vi "Find Average BP Center.vi"(7 "Tray Number":i32, 9 "XYZTheta":dbl[](array[numeric]), 11 "Gantry In":refnum<k24>) -> (1 "XYZTheta Centers":dbl[][](array[numeric]), 3 "Gantry Out":refnum<k24>)   [LabVIEW 2019, in "Assembly Tray.lvclass"]
uses:
  Assembly Tray.lvclass
  Controller/Camera/Machine Vision.ctl
  C:/Program Files (x86)/Aerotech/A3200/LabVIEW/2010/Bin/Aerotech.A3200.dll
  Program Files (x86)/Aerotech/A3200/LabVIEW/2010/Bin/Aerotech.A3200.dll
  Find Tray.ctl
  Controller/Camera/Camera.lvclass
  Controller/Motion/A3200/A3200.lvclass
panel:
  in  "Record Point 5":bool
  in  "Record Point 6":bool
  out "P5 XY":dbl[](array[numeric])
  out "P6 XY":dbl[](array[numeric])
  in  "Go to Point 5":bool
  in  "Go to Point 6":bool
  in  "Carrier Tray":T1
  in  "Go to Center":bool
  in  "Joystick":bool
  in  "Go to Syringe Area":bool
  in  "Record Syringe Area":bool
  out "Syringe Area":dbl[](array[numeric])
  out "Center":dbl[](array[numeric])
  in  "Record Point 2":bool
  in  "Record Point 3":bool
  in  "Record Point 1":bool
  in  "Record Point 4":bool
  out "P3 XY":dbl[](array[numeric])
  out "P4 XY":dbl[](array[numeric])
  out "P2 XY":dbl[](array[numeric])
  out "P1 XY":dbl[](array[numeric])
  in  "Go to Point 1":bool
  in  "Go to Point 2":bool
  in  "Go to Point 3":bool
  in  "Go to Point 4":bool
  out "Gantry":dbl[](array[numeric])
  out "Sum":dbl[](array[numeric])
  in  "Position":bool=TRUE
  in  "Stop Program":bool
  out "Image":T2(plugin-control)
  out "Camera":dbl[](array[numeric])
  in  "Machine Vision":T3=enum."Tray Fiducials"
  # "1"
  # "2"
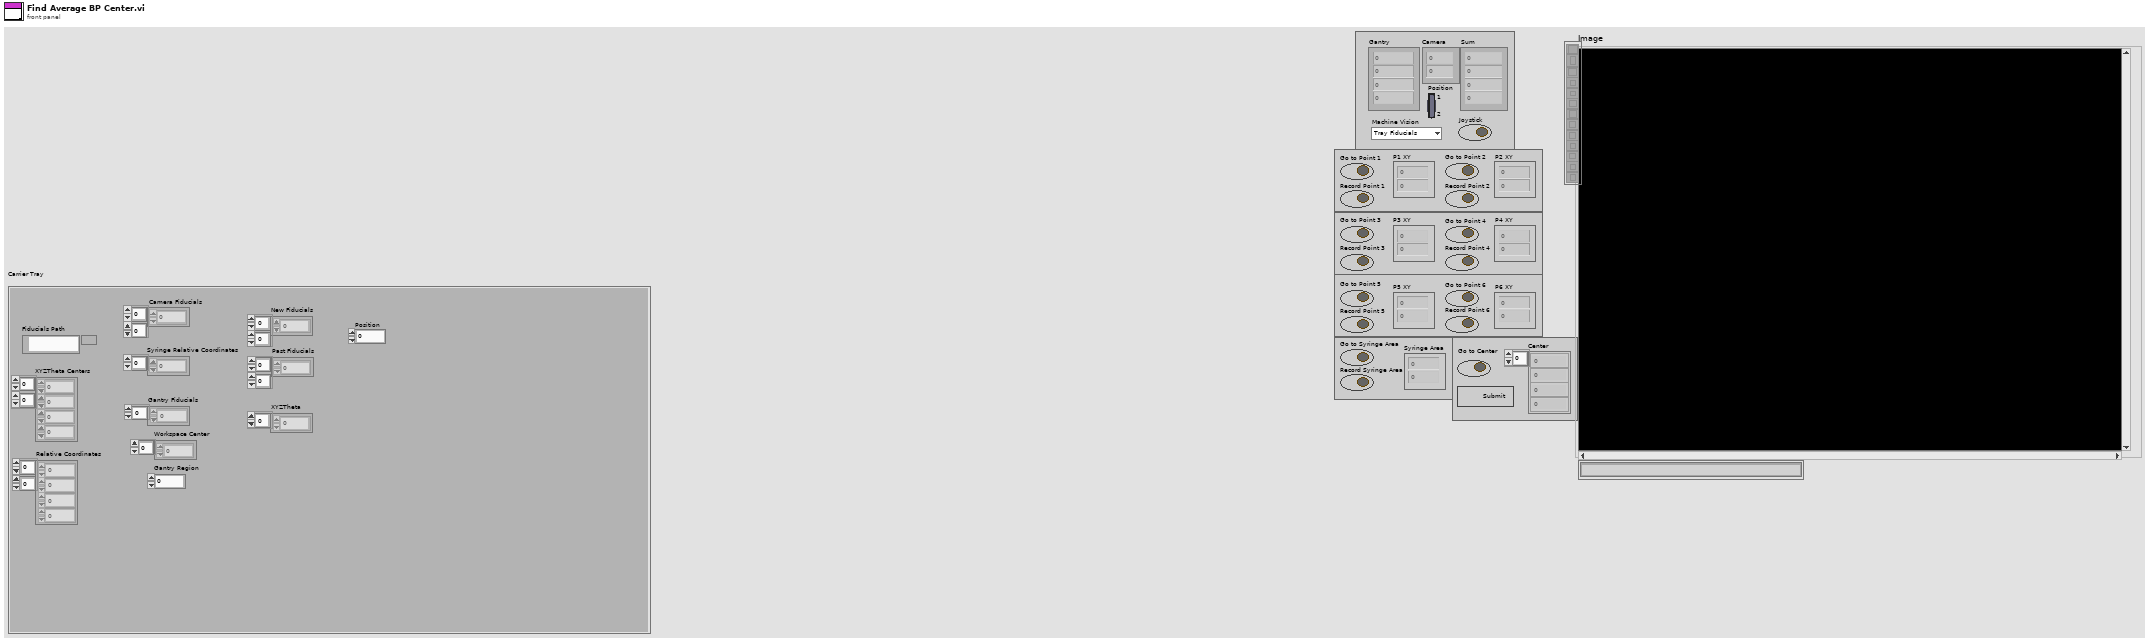
[diagram p1: front panel]
types:
  T1 = typedef "Assembly Tray.lvclass/Find Tray.ctl" = cluster{"Gantry Fiducials":dbl[], "Relative Coordinates":dbl[][], "Camera Fiducials":dbl[][], "XYZTheta Centers":dbl[][], "Workspace Center":dbl[], "Syringe Relative Coordinates":dbl[], "Gantry Region":dbl, "Fiducials Path":path, "New Fiducials":dbl[][], "Past Fiducials":dbl[][], "XYZTheta":dbl[], "Position":i32}
  T2 = typedef "IMAQ Image.ctl" = refnum<image>
  T3 = typedef "Camera.lvclass/Machine Vision.ctl" = enum16{"None", "Tray Fiducials", "HPK Silicon", "Hexaboard", "Corner (TL, BR)", "Corner (BL, TR)", "PTEG silicon TL", "PETG silicon BL", "PTEG silicon TR", "PTEG silicon BR", "PTEG PCB TL", "PTEG PCB BL", "PTEG PCB TR", "PTEG PCB BR", "dummy silicon TL", "dummy silicon BL", "dummy silicon TR", "dummy silicon BR", "dummy PCB TL", "dummy PCB BL", "dummy PCB TR", "dummy PCB BR", "baseplate TL", "baseplate BL", "baseplate TR", "baseplate BR", "BP P1", "BP P2", "BP P3", "BP P4", "BP P5", "BP P6"}
  T4 = typedef "File Paths.ctl" = cluster{"Glue Pattern Folder":path, "Carrier Tray Folder":path, "Pick Up Tool Fixture Folder":path, "Components Folder":path, "Bellows Tool Offset.txt":path, "Pick Up Tool Offset.txt":path, "Dispense Tip Offset.txt":path, "Log Files":path}
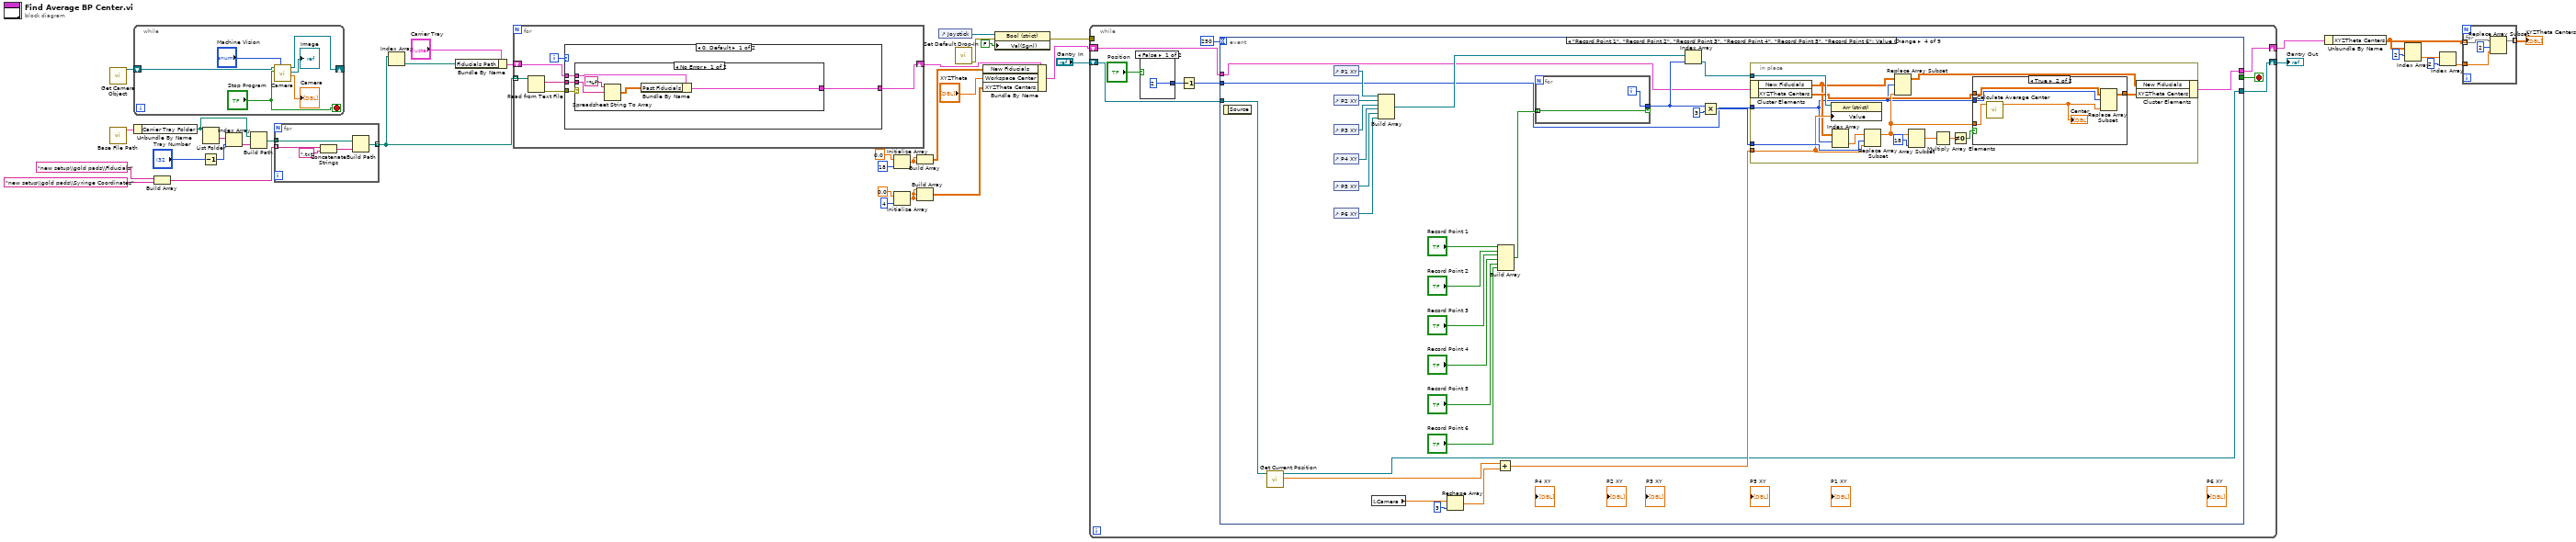
[diagram p0: block diagram]
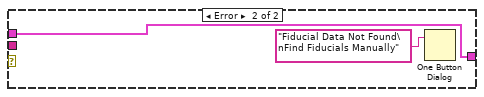
[diagram p2: hidden frame]
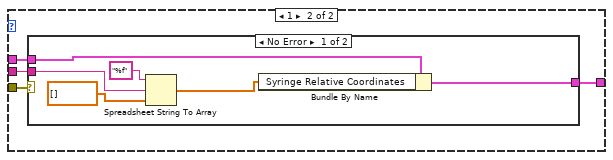
[diagram p3: hidden frame]
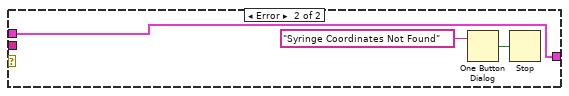
[diagram p4: hidden frame]
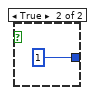
[diagram p5: hidden frame]
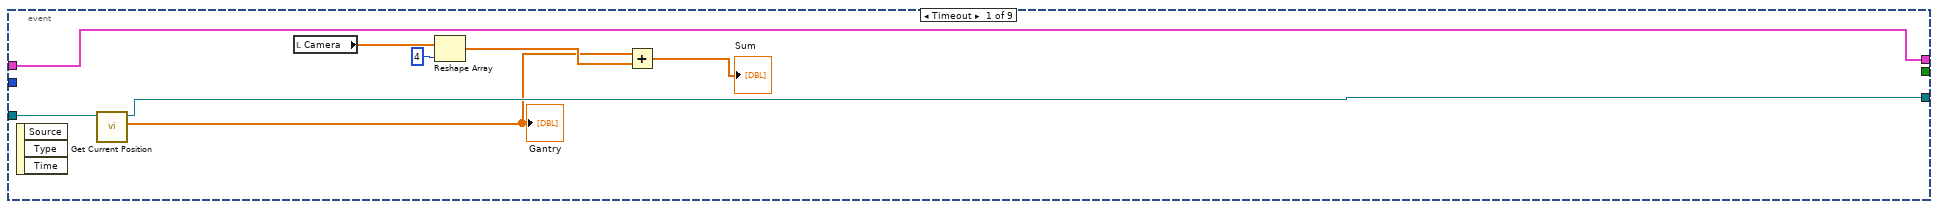
[diagram p6: hidden frame]
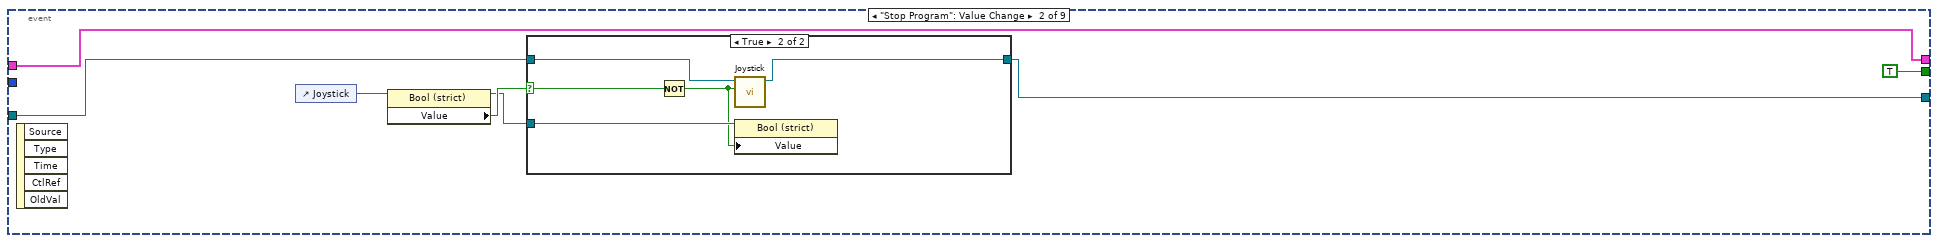
[diagram p7: hidden frame]
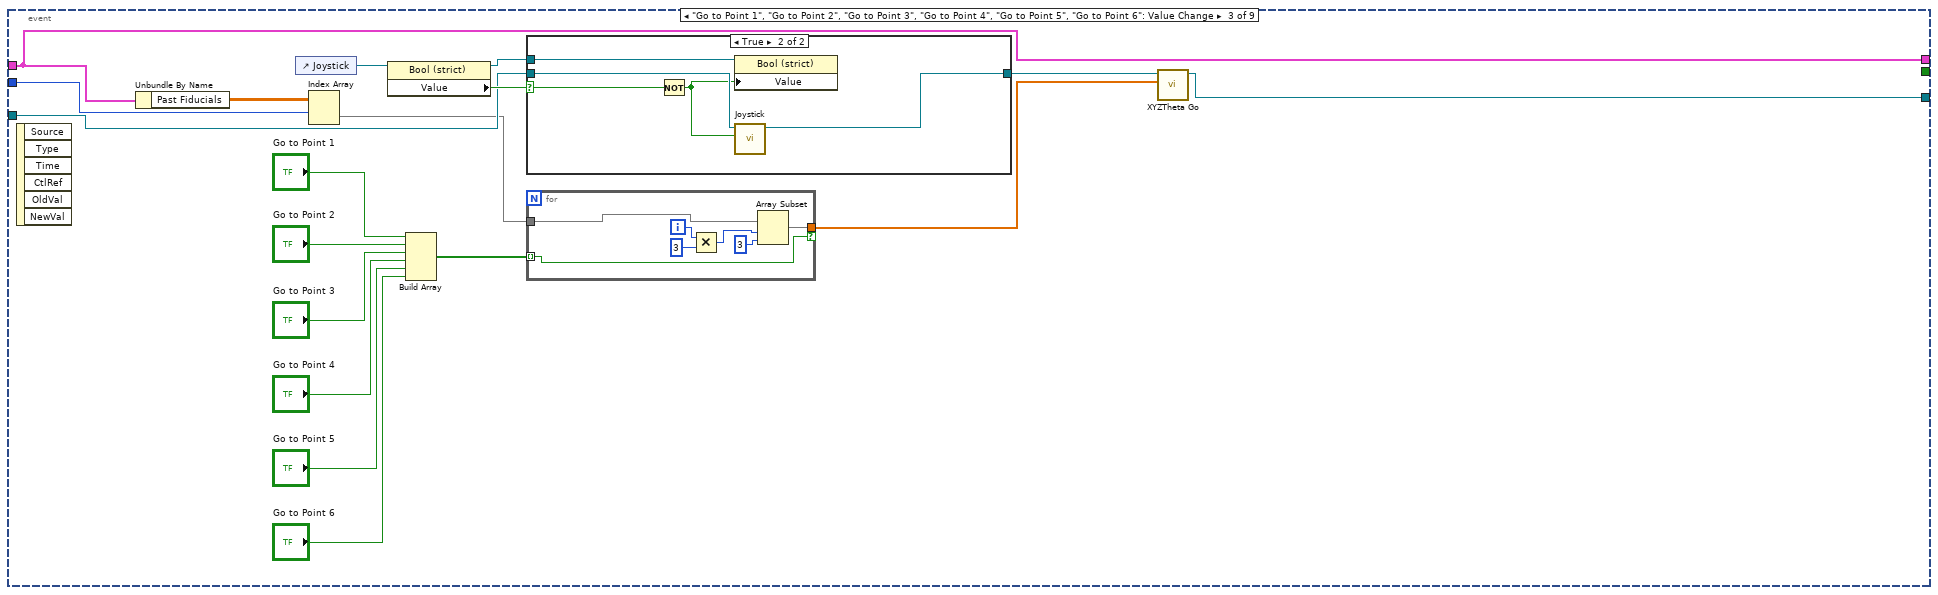
[diagram p9: hidden frame]
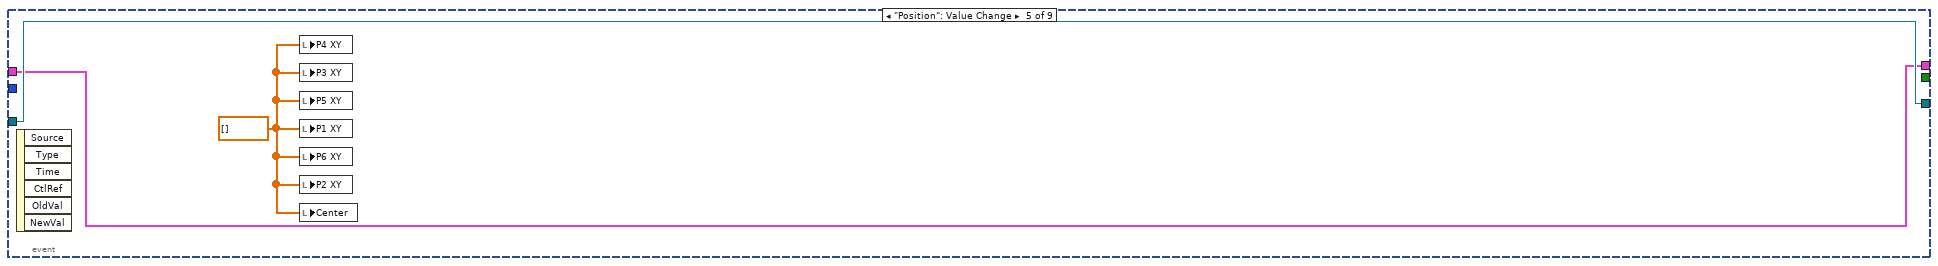
[diagram p12: hidden frame]
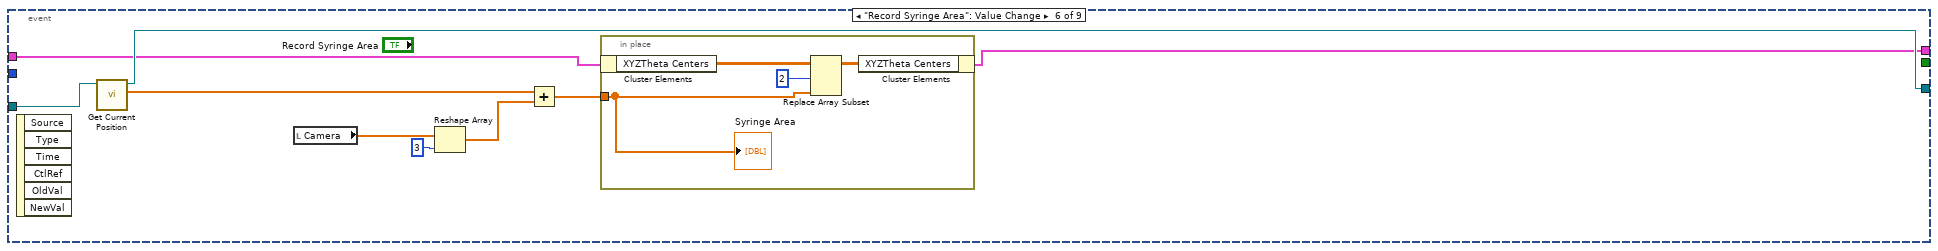
[diagram p13: hidden frame]
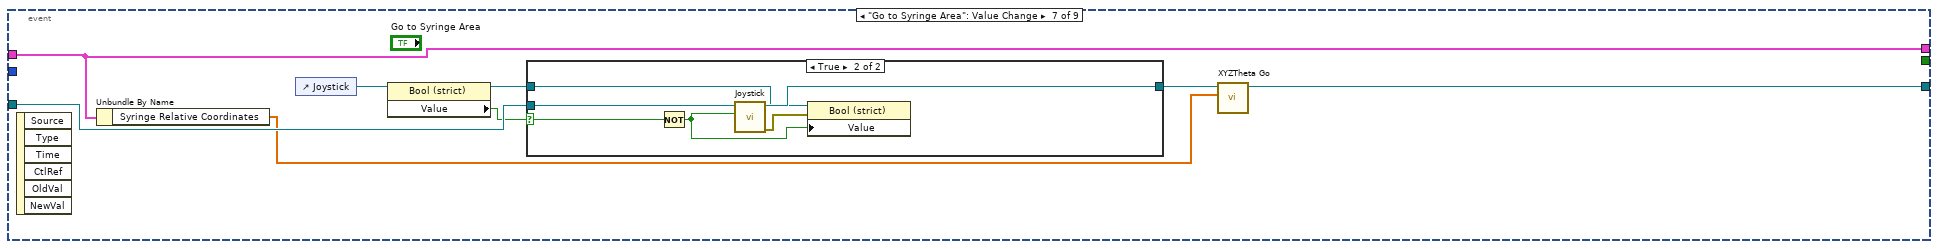
[diagram p14: hidden frame]
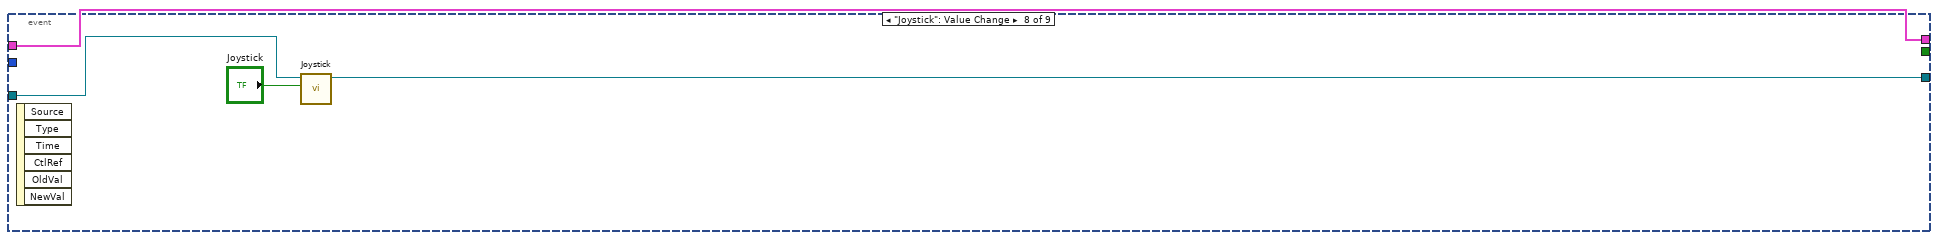
[diagram p16: hidden frame]
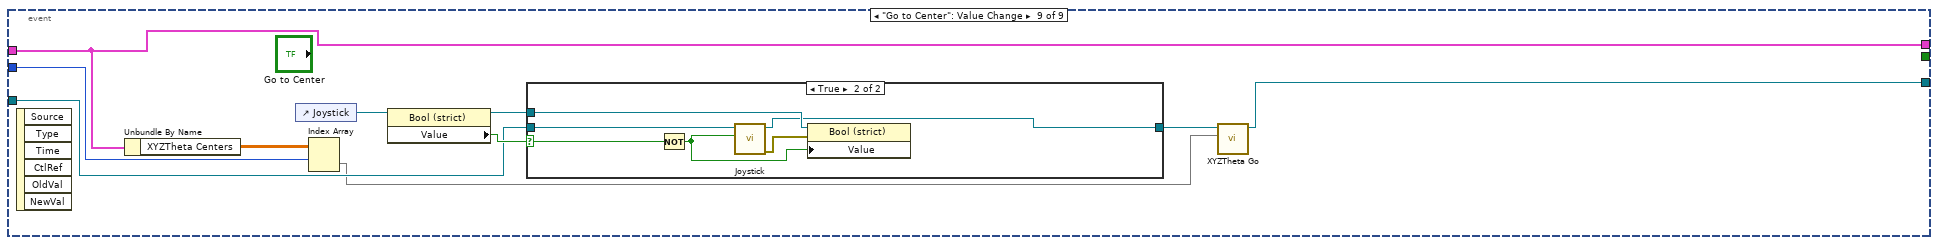
[diagram p17: hidden frame]
diagram:
  n1 = call "Get Camera Object.vi"() -> ("Camera out"=w1:refnum<class "Camera.lvclass">)  [unwired: 10 in, 1 out]
  n2 = call "Base File Path.vi"() -> ("Paths Out"=w22:T4)  [unwired: 11 in]
  n3 = while {
    shift-right: [w40] -> _
    shift-left: w1 -> [w44]
    stop <- "Stop Program" stop-if-true
    n4 = call "Camera.vi"("Machine Vision"="Machine Vision", "Stop"="Stop Program", "Camera in"=w44) -> ("Camera"=→"Camera":dbl[], "Image"=→"Image":T2, "Camera out"=w40:refnum<class "Camera.lvclass">)  [unwired: 5 in, 1 out]
  }
  n5 = Unbundle By Name(w22) -> ("Carrier Tray Folder"=w20:path)
  n6 = Build Array("new setup\\gold pads\\Fiducials" ("format string"), "new setup\\gold pads\\Syringe Coordinates" ("element")) -> (w25:string[])
  n7 = Decrement(x="Tray Number") -> (x-1=w21:i32)
  n8 = List Folder(path=w20) -> (folder names=w24:string[])  [unwired: 3 in, 3 out]
  n9 = Index Array(array=w24, index=w21) -> (element=w23:string)
  n10 = Build Path(base path=w20, name or relative path=w23) -> (appended path=w26:path)
  n11 = for {
    tunnel: w25 -> [w48] mode=indexing
    tunnel: w26 -> [w50]
    tunnel: [w49] -> w19 mode=indexing
    n12 = Concatenate Strings(w48, ".txt" ("string")) -> (w46:string)
    n13 = Build Path(base path=w50, name or relative path=w46) -> (appended path=w49:path)
  }
  n14 = Index Array(array=w19) -> (element=w27:path)  [unwired: 1 in]
  n15 = Bundle By Name(cluster="Carrier Tray", "Fiducials Path"=w27) -> (w29:T1)
  n16 = for {
    tunnel: w19 -> [w55] mode=indexing
    shift-right: [w51] -> w16
    shift-left: w29 -> [w52]
    i -> [w53]
    n17 = Read from Text File(file (use dialog)=w55) -> (text=w56:string, error out=w54:errorcluster)  [unwired: 3 in, 2 out]
    n18 = case shown="0, Default" w53 {
      tunnel: w56 -> [w60 w69]
      tunnel: w54 -> [w59 w70]
      tunnel: w52 -> [w58 w71]
      tunnel: [w57 w68] -> w51
      frame 0, Default {
        n19 = case shown="No Error" w59 {
          tunnel: w60 -> [w64 _]
          tunnel: w58 -> [w62 w66]
          tunnel: [w63 w66] -> w57
          frame No Error {
            n20 = Spreadsheet String To Array(format string="%f", spreadsheet string=w64) -> (array=w61:dbl[][])  [unwired: 2 in]
            n21 = Bundle By Name(cluster=w62, "Past Fiducials"=w61) -> (w63:T1)
          }
          frame Error {
            n22 = One Button Dialog(message="Fiducial Data Not Found\nFind Fiducials Manually") -> ()  [unwired: 1 in, 1 out]
          }
        }
      }
      frame 1 {
        n23 = case shown="No Error" w70 {
          tunnel: w69 -> [w75 _]
          tunnel: [w73 w78] -> w68
          tunnel: w71 -> [w74 w78]
          frame No Error {
            n24 = Spreadsheet String To Array(format string="%f", spreadsheet string=w75, array type (2D Dbl)=dbl[] []) -> (array=w72:dbl[])  [unwired: 1 in]
            n25 = Bundle By Name(cluster=w74, "Syringe Relative Coordinates"=w72) -> (w73:T1)
          }
          frame Error {
            n26 = One Button Dialog(message="Syringe Coordinates Not Found") -> (true=w79:bool)  [unwired: 1 in]
            n27 = Stop(stop? (T)=w79) -> ()
          }
        }
      }
    }
  }
  n28 = Initialize Array(0.0 ("element"), 18 ("dimension size")) -> (w13:dbl[])
  n29 = Initialize Array(0.0 ("element"), 4 ("dimension size")) -> (w9:dbl[])
  n30 = Build Array(w13, w13) -> (w14:dbl[][])
  n31 = Build Array(w9, w9, w9) -> (w8:dbl[][])
  n32 = control-ref of="Joystick"() -> (w38:refnum<vi>)
  n33 = call "Set Default Drop-In.vi"() -> ("error out"=w32:errorcluster)  [unwired: 11 in]
  n34 = Bundle By Name(cluster=w16, "New Fiducials"=w14, "Workspace Center"="XYZTheta", "XYZTheta Centers"=w8) -> (w39:T1)
  n35 = property class="Bool (strict)"(reference=w38, error in=w32, "Val(Sgnl)"=FALSE) -> (error out=w36:errorcluster)  [unwired: 1 out]
  n36 = while {
    shift-right: [w81] -> w12
    shift-left: w39 -> [w88]
    tunnel: w36 -> [_]
    shift-right: [w85] -> w30
    shift-left: "Gantry In" -> [w86]
    stop <- w89 stop-if-true
    n37 = case shown="False" "Position" {
      tunnel: [2 1] -> w82
      frame False {
      }
      frame True {
      }
    }
    n38 = Decrement(x=w82) -> (x-1=w84:i32)
    n39 = event shown="[3] \"Record Point 1\", \"Record Point 2\", \"Record Point 3\", \"Record Point 4\", \"Record Point 5\", \"Record Point 6\": Value Change" {
      selector: _ -> [_ _ _ _ _ _ _ _ _]
      dyn-events: _ -> [_ _ _ _ _ _ _ _ _]
      timeout: 250 -> [_ _ _ _ _ _ _ _ _]
      tunnel: [_ TRUE _ _ _ _ _ _ _] -> w89
      tunnel: w88 -> [w98 w101 w124 w149 w195 w199 w217 w228 w238]
      tunnel: [w98 w101 w124 w171 w195 w198 w217 w228 w238] -> w81
      tunnel: w86 -> [w94 w102 w121 w152 w196 w205 w214 w227 w234]
      tunnel: [w93 w100 w118 w150 w196 w200 w216 w225 w232] -> w85
      tunnel: w84 -> [_ _ w115 w148 _ _ _ _ w230]
      event Timeout {
        n40 = event-data() -> ()  [unwired: 1 in, 3 out]
        n41 = call "Get Current Position.vi"("Gantry In"=w94) -> ("XYZTheta Out"=w92:dbl[], "Gantry Out"=w93:refnum<k24>)  [unwired: 8 in, 1 out]
        "Gantry" <- w92
        n42 = local read "Camera"() -> (w97:dbl[])
        n43 = Reshape Array(w97, 4 ("dimension size")) -> (w95:dbl[])
        n44 = Add(x=w92, y=w95) -> (x+y=→"Sum":dbl[])
      }
      event "Stop Program": Value Change {
        n45 = event-data() -> ()  [unwired: 1 in, 5 out]
        n46 = control-ref of="Joystick"() -> (w103:refnum<vi>)
        n47 = property class="Bool (strict)"(reference=w103) -> (reference out=w104:refnum<vi>, "Value"=w105:bool)  [unwired: 1 in, 1 out]
        n48 = case shown="True" w105 {
          selector: w105 -> [_ w112]
          tunnel: w102 -> [w107 w110]
          tunnel: [w107 w109] -> w100
          tunnel: w104 -> [_ w111]
          frame False {
          }
          frame True {
            n49 = Not(x=w112) -> (.not. x?=w108:bool)
            n50 = call "Joystick.vi"("Joystick"=w108, "Gantry In"=w110) -> ("Gantry Out"=w109:refnum<k24>)  [unwired: 8 in, 1 out]
            n51 = property class="Bool (strict)"(reference=w111, "Value"=w108) -> ()  [unwired: 1 in, 2 out]
          }
        }
      }
      event "Go to Point 1", "Go to Point 2", "Go to Point 3", "Go to Point 4", "Go to Point 5", "Go to Point 6": Value Change {
        n52 = event-data() -> ()  [unwired: 1 in, 6 out]
        n53 = Unbundle By Name(w124) -> ("Past Fiducials"=w117:dbl[][])
        n54 = control-ref of="Joystick"() -> (w119:refnum<vi>)
        n55 = Index Array(array=w117, index (row)=w115) -> (element=w116:dbl[])  [unwired: 1 in]
        n56 = property class="Bool (strict)"(reference=w119) -> (reference out=w122:refnum<vi>, "Value"=w123:bool)  [unwired: 1 in, 1 out]
        n57 = Build Array("Go to Point 1", "Go to Point 2", "Go to Point 3", "Go to Point 4", "Go to Point 5", "Go to Point 6") -> (w126:bool[])
        n58 = case shown="True" w123 {
          selector: w123 -> [_ w136]
          tunnel: w121 -> [w131 w134]
          tunnel: [w131 w132] -> w120
          tunnel: w122 -> [_ w135]
          frame False {
          }
          frame True {
            n59 = Not(x=w136) -> (.not. x?=w133:bool)
            n60 = property class="Bool (strict)"(reference=w135, "Value"=w133) -> ()  [unwired: 1 in, 2 out]
            n61 = call "Joystick.vi"("Joystick"=w133, "Gantry In"=w134) -> ("Gantry Out"=w132:refnum<k24>)  [unwired: 8 in, 1 out]
          }
        }
        n62 = for {
          tunnel: w126 -> [w143] mode=indexing
          tunnel: w116 -> [w142]
          tunnel: [w137] -> w125 if=w143
          i -> [w140]
          n63 = Multiply(x=w140, y=3) -> (x*y=w138:i32)
          n64 = Array Subset(array=w142, index=w138, length=3) -> (w137:dbl[])
        }
        n65 = call "XYZTheta Go.vi"("XYZTheta In"=w125, "Gantry In"=w120) -> ("Gantry Out"=w118:refnum<k24>)  [unwired: 7 in, 2 out]
      }
      event "Record Point 1", "Record Point 2", "Record Point 3", "Record Point 4", "Record Point 5", "Record Point 6": Value Change {
        n66 = event-data() -> ()  [unwired: 1 in, 1 out]
        n67 = call "Get Current Position.vi"("Gantry In"=w152) -> ("XYZTheta Out"=w151:dbl[], "Gantry Out"=w150:refnum<k24>)  [unwired: 8 in, 1 out]
        n68 = control-ref of="P1 XY"() -> (w165:refnum<vi>)
        n69 = control-ref of="P2 XY"() -> (w164:refnum<vi>)
        n70 = control-ref of="P3 XY"() -> (w163:refnum<vi>)
        n71 = control-ref of="P4 XY"() -> (w162:refnum<vi>)
        n72 = control-ref of="P5 XY"() -> (w145:refnum<vi>)
        n73 = control-ref of="P6 XY"() -> (w144:refnum<vi>)
        n74 = local read "Camera"() -> (w155:dbl[])
        n75 = Build Array(w165, w164, w163, w162, w145, w144) -> (w161:refnum<vi>[])
        n76 = Reshape Array(w155, 3 ("dimension size")) -> (w154:dbl[])
        n77 = Add(x=w151, y=w154) -> (x+y=w153:dbl[])
        n78 = Build Array("Record Point 1", "Record Point 2", "Record Point 3", "Record Point 4", "Record Point 5", "Record Point 6") -> (w166:bool[])
        n79 = for {
          tunnel: w166 -> [w172] mode=indexing
          tunnel: [w173] -> w158 if=w172
          i -> [w173]
        }
        n80 = Index Array(array=w161, index=w158) -> (element=w160:refnum<vi>)
        n81 = Multiply(x=w158, y=3) -> (x*y=w156:i32)
        n82 = in-place {
          in-place-border: w156 -> [w187]
          in-place-border: w160 -> [w185]
          in-place-border: w153 -> [w184]
          in-place-border: w148 -> [w175]
          n83 = in-place-cluster #1(w149) -> ("New Fiducials"=w176:dbl[][], "XYZTheta Centers"=w178:dbl[][])
          n84 = property class="Arr (strict)"(reference=w185, "Value"=w184) -> ()  [unwired: 1 in, 2 out]
          n85 = Index Array(array=w176, index (row)=w175) -> (element=w179:dbl[])  [unwired: 1 in]
          n86 = Replace Array Subset(array=w179, new element=w184, index=w187) -> (w183:dbl[])
          n87 = Replace Array Subset(array=w176, new element=w183, index (row)=w175) -> (w174:dbl[][])  [unwired: 1 in]
          n88 = Array Subset(array=w183, length=18) -> (w181:dbl[])  [unwired: 1 in]
          n89 = Multiply Array Elements(1:w181) -> (0:w180:dbl)
          n90 = Not Equal To 0?(x=w180) -> (x != 0?=w186:bool)
          n91 = case shown="True" w186 {
            tunnel: w183 -> [_ w190]
            tunnel: w178 -> [w188 w192]
            tunnel: w175 -> [_ w189]
            tunnel: [w188 w191] -> w177
            frame False {
            }
            frame True {
              n92 = call "Calculate Average Center.vi"("Gantry Fiducials"=w190) -> ("XYZTheta"=w193:dbl[])  [unwired: 10 in]
              "Center" <- w193
              n93 = Replace Array Subset(array=w192, new element=w193, index (row)=w189) -> (w191:dbl[][])  [unwired: 1 in]
            }
          }
          n94 = in-place-cluster #1("New Fiducials"=w174, "XYZTheta Centers"=w177) -> (w171:T1)
        }
      }
      event "Position": Value Change {
        w194 = dbl[] [] ("TR XY")
        n95 = event-data() -> ()  [unwired: 1 in, 6 out]
        n96 = local write "P4 XY"(w194) -> ()
        n97 = local write "P3 XY"(w194) -> ()
        n98 = local write "P5 XY"(w194) -> ()
        n99 = local write "P1 XY"(w194) -> ()
        n100 = local write "P6 XY"(w194) -> ()
        n101 = local write "P2 XY"(w194) -> ()
        n102 = local write "Center"(w194) -> ()
      }
      event "Record Syringe Area": Value Change {
        n103 = event-data() -> ()  [unwired: 1 in, 6 out]
        n104 = call "Get Current Position.vi"("Gantry In"=w205) -> ("XYZTheta Out"=w201:dbl[], "Gantry Out"=w200:refnum<k24>)  [unwired: 8 in, 1 out]
        n105 = local read "Camera"() -> (w202:dbl[])
        n106 = Reshape Array(w202, 3 ("dimension size")) -> (w203:dbl[])
        n107 = Add(x=w201, y=w203) -> (x+y=w197:dbl[])
        n108 = in-place {
          in-place-border: w197 -> [w208]
          n109 = in-place-cluster #2(w199) -> ("XYZTheta Centers"=w209:dbl[][])
          n110 = Replace Array Subset(array=w209, new element=w208, index (row)=2) -> (w206:dbl[][])  [unwired: 1 in]
          n111 = in-place-cluster #2("XYZTheta Centers"=w206) -> (w198:T1)
          "Syringe Area" <- w208
        }
      }
      event "Go to Syringe Area": Value Change {
        n112 = event-data() -> ()  [unwired: 1 in, 6 out]
        n113 = Unbundle By Name(w217) -> ("Syringe Relative Coordinates"=w210:dbl[])
        n114 = control-ref of="Joystick"() -> (w213:refnum<vi>)
        n115 = property class="Bool (strict)"(reference=w213) -> (reference out=w211:refnum<vi>, "Value"=w212:bool)  [unwired: 1 in, 1 out]
        n116 = case shown="True" w212 {
          selector: w212 -> [_ w220]
          tunnel: [w218 w224] -> w215
          tunnel: w214 -> [w218 w223]
          tunnel: w211 -> [_ w222]
          frame False {
          }
          frame True {
            n117 = Not(x=w220) -> (.not. x?=w219:bool)
            n118 = call "Joystick.vi"("Joystick"=w219, "Gantry In"=w223) -> ("error out"=w221:errorcluster, "Gantry Out"=w224:refnum<k24>)  [unwired: 8 in]
            n119 = property class="Bool (strict)"(reference=w222, error in=w221, "Value"=w219) -> ()  [unwired: 2 out]
          }
        }
        n120 = call "XYZTheta Go.vi"("XYZTheta In"=w210, "Gantry In"=w215) -> ("Gantry Out"=w216:refnum<k24>)  [unwired: 7 in, 2 out]
      }
      event "Joystick": Value Change {
        n121 = event-data() -> ()  [unwired: 1 in, 6 out]
        n122 = call "Joystick.vi"("Joystick"="Joystick", "Gantry In"=w227) -> ("Gantry Out"=w225:refnum<k24>)  [unwired: 8 in, 1 out]
      }
      event "Go to Center": Value Change {
        n123 = event-data() -> ()  [unwired: 1 in, 6 out]
        n124 = Unbundle By Name(w238) -> ("XYZTheta Centers"=w231:dbl[][])
        n125 = control-ref of="Joystick"() -> (w235:refnum<vi>)
        n126 = Index Array(array=w231, index (row)=w230) -> (element=w229:dbl[])  [unwired: 1 in]
        n127 = property class="Bool (strict)"(reference=w235) -> (reference out=w236:refnum<vi>, "Value"=w237:bool)  [unwired: 1 in, 1 out]
        n128 = case shown="True" w237 {
          selector: w237 -> [_ w245]
          tunnel: w234 -> [w239 w242]
          tunnel: [w239 w241] -> w233
          tunnel: w236 -> [_ w244]
          frame False {
          }
          frame True {
            n129 = Not(x=w245) -> (.not. x?=w240:bool)
            n130 = call "Joystick.vi"("Joystick"=w240, "Gantry In"=w242) -> ("error out"=w243:errorcluster, "Gantry Out"=w241:refnum<k24>)  [unwired: 8 in]
            n131 = property class="Bool (strict)"(reference=w244, error in=w243, "Value"=w240) -> ()  [unwired: 2 out]
          }
        }
        n132 = call "XYZTheta Go.vi"("XYZTheta In"=w229, "Gantry In"=w233) -> ("Gantry Out"=w232:refnum<k24>)  [unwired: 7 in, 2 out]
      }
    }
  }
  "Gantry Out" <- w30
  n133 = Unbundle By Name(w12) -> ("XYZTheta Centers"=w4:dbl[][])
  n134 = Index Array(array=w4, index (row)=2) -> (element=w6:dbl[])  [unwired: 1 in]
  n135 = Index Array(array=w6, index=2) -> (element=w3:dbl)
  n136 = for {
    tunnel: w4 -> [w249] mode=indexing
    tunnel: w3 -> [w248]
    tunnel: [w247] -> w2 mode=indexing
    n137 = Replace Array Subset(array=w249, new element=w248, index=2) -> (w247:dbl[])
  }
  "XYZTheta Centers" <- w2
